vi "JSON Object Deltas.vi"(6 "index  offset":i32, 7 "name":string, 8 "delta index":i32, 9 "delta tokens":cluster{"token type":T3, "Type Definition":T4}[](array[cluster]), 10 "full index":i32, 11 "full tokens":cluster{"token type":T3, "Type Definition":T4}[](array[cluster])) -> (3 "Subs":T1(array[cluster]))   [LabVIEW 2019]
uses:
  <vilib>/MultiError/TokenizeJSON/Multi Error Cluster.lvlib
  <vilib>/MultiError/TokenizeJSON/JSON Token Values.ctl
  <vilib>/MultiError/TokenizeJSON/JSON Raw Token Values.ctl
  <vilib>/MultiError/Errors Cluster Multiple Errors/JSON Token Descriptor.ctl
panel:
  out "Output":T2(array[cluster])
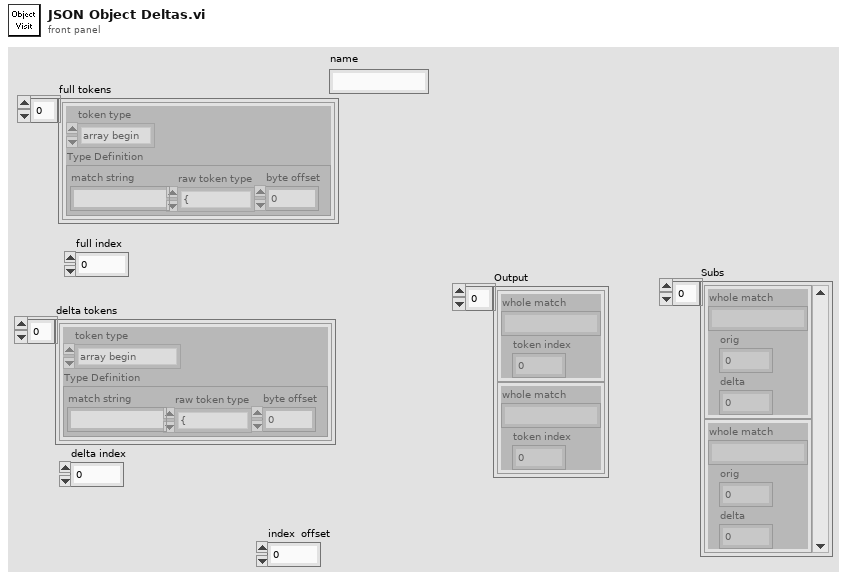
[diagram p1: front panel]
types:
  T1 = cluster{"whole match":string, "orig":i32, "delta":i32}[]
  T2 = cluster{"whole match":string, "token index":i32}[]
  T3 = typedef "Multi Error Cluster.lvlib/JSON Token Values.ctl" = enum32{"array begin", "array end", "object begin", "object end", "value", "invalid", "name"}
  T4 = typedef "Multi Error Cluster.lvlib/JSON Token Descriptor.ctl" = cluster{"match string":string, "raw token type":T5, "byte offset ":i32}
  T5 = typedef "Multi Error Cluster.lvlib/JSON Raw Token Values.ctl" = enum32{"{", "}", "[", "]", ",", ":", "\"", "number", "string", "true", "false", "null", "invalid"}
  T6 = typedef "Multi Error Cluster.lvlib/JSON Object Descriptor.ctl" = cluster{"begin info":T4, "end info":T4, "begin Index":i32, "end Index":i32}
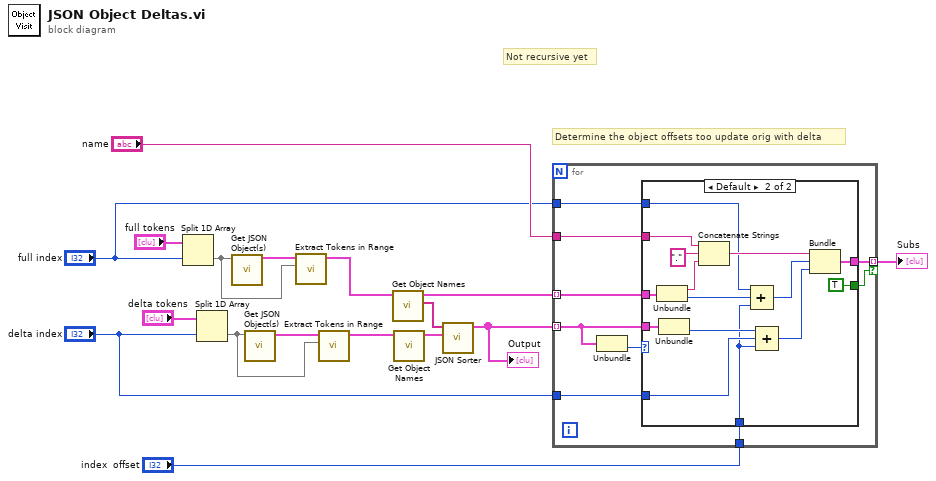
[diagram p0: block diagram]
diagram:
  # "Not recursive yet"
  # "Determine the object offsets too update orig with delta"
  n1 = Split 1D Array(array="full tokens", index="full index") -> (second subarray=w14:cluster{"token type":T3, "Type Definition":T4}[])  [unwired: 1 out]
  n2 = Split 1D Array(array="delta tokens", index="delta index") -> (second subarray=w11:cluster{"token type":T3, "Type Definition":T4}[])  [unwired: 1 out]
  n3 = call <vilib>:"Get JSON Object(s).vi"("tokens"=w14) -> ("array of JSON objects"=w13:T6[])  [unwired: 10 in]
  n4 = call <vilib>:"Get JSON Object(s).vi"("tokens"=w11) -> ("array of JSON objects"=w12:T6[])  [unwired: 10 in]
  n5 = call <vilib>:"Extract Tokens in Range.vi"("tokens"=w14, "range info"=w13) -> ("tokens out"=w10:cluster{"token type":T3, "info":T4}[])  [unwired: 9 in]
  n6 = call <vilib>:"Extract Tokens in Range.vi"("tokens"=w11, "range info"=w12) -> ("tokens out"=w9:cluster{"token type":T3, "info":T4}[])  [unwired: 9 in]
  n7 = call "Get Object Names.vi"("tokens in"=w10) -> ("Names"=w7:string[], "Array"=w5:cluster{"match string":string, i32}[])  [unwired: 9 in]
  n8 = call "Get Object Names.vi"("tokens in"=w9) -> ("Array"=w8:cluster{"match string":string, i32}[])  [unwired: 9 in, 1 out]
  n9 = call "JSON Sorter.vi"("Found Token Info"=w8, "names"=w7) -> ("Output"=w6:T2)  [unwired: 9 in]
  "Output" <- w6
  n10 = for {
    tunnel: "name" -> [w26]
    tunnel: [w25] -> w4 mode=indexing if=w23
    tunnel: w6 -> [w22] mode=indexing
    tunnel: w5 -> [w24] mode=indexing
    tunnel: "full index" -> [w20]
    tunnel: "delta index" -> [w19]
    tunnel: "index  offset" -> [w18]
    n11 = Unbundle(w22) -> ("token index"=w21:i32)  [unwired: 1 out]
    n12 = case shown="Default" w21 {
      tunnel: w26 -> [_ w34]
      tunnel: [_ w41] -> w25
      tunnel: w22 -> [_ w40]
      tunnel: w24 -> [_ w39]
      tunnel: [_ TRUE] -> w23
      tunnel: w20 -> [_ w30]
      tunnel: w19 -> [_ w33]
      tunnel: w18 -> [_ w27]
      frame -1 {
      }
      frame Default {
        n13 = Unbundle(w39) -> ("match string"=w36:string, w29:i32)
        n14 = Unbundle(w40) -> ("token index"=w32:i32)  [unwired: 1 out]
        n15 = Concatenate Strings(w34, ".", w36) -> (w35:string)
        n16 = Compound Arithmetic op=ADD(w30, w29, w27) -> (w28:i32)
        n17 = Compound Arithmetic op=ADD(w32, w33, w27) -> (w31:i32)
        n18 = Bundle(w35, w28, w31) -> (w41:cluster{string, i32, i32})  [unwired: 1 in]
      }
    }
  }
  "Subs" <- w4
